vi "华为UPS2000-G获取UPS状态.vi"(8 "error in (no error)":errorcluster, 11 "MB session in":refnum<class "MB_Master.lvclass">) -> (0 "error out":errorcluster, 1 "UPS状态":bool[](array[boolean]), 2 "UPS参数":T1 {"开机状态" items=["关机", "开机中", "开机失败", "开机完成"]}, 3 "MB session out":refnum<class "MB_Master.lvclass">)   [LabVIEW 2016, in "环境动力监测库.lvlib" / "UPS库.lvlib"]
uses:
  <vilib>/Plasmionique/MB Master/MB_Master/MB_Master.lvclass
  <vilib>/Plasmionique/MB Master/MB Master.lvlib
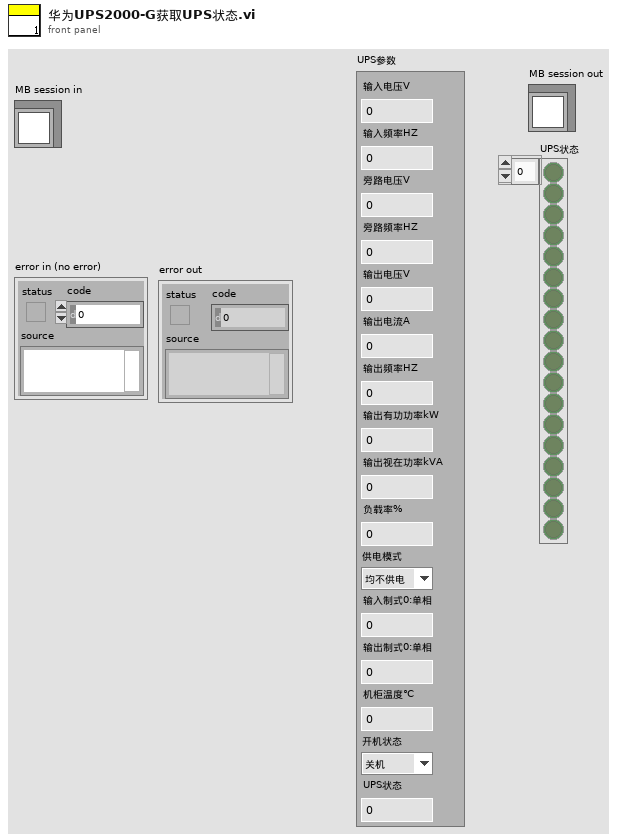
[diagram p1: front panel]
types:
  T1 = cluster{"输入电压V":dbl, "输入频率HZ":dbl, "旁路电压V":dbl, "旁路频率HZ":dbl, "输出电压V":dbl, "输出电流A":dbl, "输出频率HZ":dbl, "输出有功功率kW":dbl, "输出视在功率kVA":dbl, "负载率%":dbl, "供电模式":enum16{"均不供电", "旁路供电", "主路供电", "电池供电", "主路ECO"}, "输入制式0:单相":u16, "输出制式0:单相":u16, "机柜温度℃":dbl, "开机状态":u16, "UPS状态":u8}
  T2 = cluster{dbl, dbl, dbl, dbl, dbl, dbl, dbl, dbl, dbl, dbl, u16, u16, u16, dbl, u16, "元素":u16}
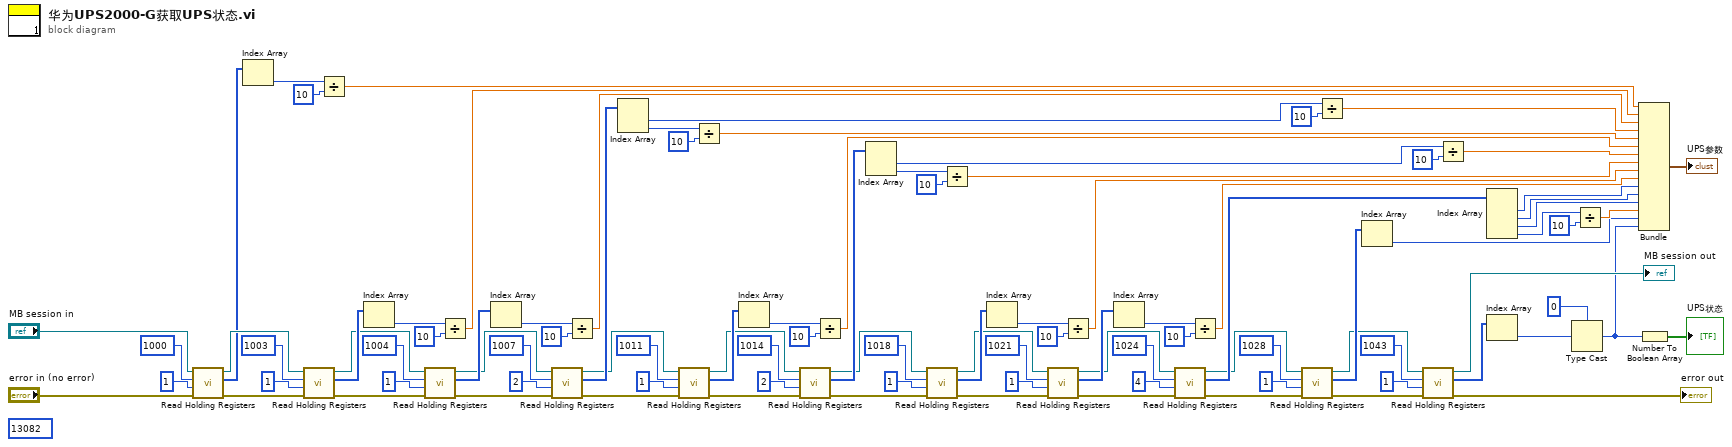
[diagram p0: block diagram]
diagram:
  (unwired) u16 13082 ("starting address")
  n1 = call <vilib>:"Read Holding Registers.vi"("error in (no error)"="error in (no error)", "quantity"=u16 1, "starting address"=u16 1000, "MB session in"="MB session in") -> ("error out"=w87:errorcluster, "Registers"=w93:u16[], "MB session out"=w96:refnum<class "MB_Master.lvclass">)  [unwired: 5 in]
  n2 = Index Array(array=w93) -> (element=w91:u16)  [unwired: 1 in]
  n3 = call <vilib>:"Read Holding Registers.vi"("error in (no error)"=w87, "quantity"=u16 1, "starting address"=u16 1003, "MB session in"=w96) -> ("error out"=w79:errorcluster, "Registers"=w84:u16[], "MB session out"=w80:refnum<class "MB_Master.lvclass">)  [unwired: 5 in]
  n4 = Divide(x=w91, y=u16 10) -> (x/y=w90:dbl)
  n5 = Index Array(array=w84) -> (element=w86:u16)  [unwired: 1 in]
  n6 = call <vilib>:"Read Holding Registers.vi"("error in (no error)"=w79, "quantity"=u16 1, "starting address"=u16 1004, "MB session in"=w80) -> ("error out"=w71:errorcluster, "Registers"=w76:u16[], "MB session out"=w72:refnum<class "MB_Master.lvclass">)  [unwired: 5 in]
  n7 = Divide(x=w86, y=u16 10) -> (x/y=w83:dbl)
  n8 = Index Array(array=w76) -> (element=w77:u16)  [unwired: 1 in]
  n9 = call <vilib>:"Read Holding Registers.vi"("error in (no error)"=w71, "quantity"=u16 2, "starting address"=u16 1007, "MB session in"=w72) -> ("error out"=w60:errorcluster, "Registers"=w68:u16[], "MB session out"=w61:refnum<class "MB_Master.lvclass">)  [unwired: 5 in]
  n10 = Divide(x=w77, y=u16 10) -> (x/y=w75:dbl)
  n11 = Index Array(array=w68) -> (element #1=w70:u16, element #2=w66:u16)  [unwired: 2 in]
  n12 = call <vilib>:"Read Holding Registers.vi"("error in (no error)"=w60, "quantity"=u16 1, "starting address"=u16 1011, "MB session in"=w61) -> ("error out"=w52:errorcluster, "Registers"=w57:u16[], "MB session out"=w53:refnum<class "MB_Master.lvclass">)  [unwired: 5 in]
  n13 = Divide(x=w66, y=u16 10) -> (x/y=w64:dbl)
  n14 = Index Array(array=w57) -> (element=w59:u16)  [unwired: 1 in]
  n15 = call <vilib>:"Read Holding Registers.vi"("error in (no error)"=w52, "quantity"=u16 2, "starting address"=u16 1014, "MB session in"=w53) -> ("error out"=w41:errorcluster, "Registers"=w50:u16[], "MB session out"=w42:refnum<class "MB_Master.lvclass">)  [unwired: 5 in]
  n16 = Divide(x=w59, y=u16 10) -> (x/y=w56:dbl)
  n17 = Index Array(array=w50) -> (element #1=w51:u16, element #2=w47:u16)  [unwired: 2 in]
  n18 = call <vilib>:"Read Holding Registers.vi"("error in (no error)"=w41, "quantity"=u16 1, "starting address"=u16 1018, "MB session in"=w42) -> ("error out"=w33:errorcluster, "Registers"=w39:u16[], "MB session out"=w35:refnum<class "MB_Master.lvclass">)  [unwired: 5 in]
  n19 = Divide(x=w47, y=u16 10) -> (x/y=w45:dbl)
  n20 = Index Array(array=w39) -> (element=w40:u16)  [unwired: 1 in]
  n21 = call <vilib>:"Read Holding Registers.vi"("error in (no error)"=w33, "quantity"=u16 1, "starting address"=u16 1021, "MB session in"=w35) -> ("error out"=w25:errorcluster, "Registers"=w31:u16[], "MB session out"=w26:refnum<class "MB_Master.lvclass">)  [unwired: 5 in]
  n22 = Divide(x=w40, y=u16 10) -> (x/y=w34:dbl)
  n23 = Index Array(array=w31) -> (element=w37:u16)  [unwired: 1 in]
  n24 = call <vilib>:"Read Holding Registers.vi"("error in (no error)"=w25, "quantity"=u16 4, "starting address"=u16 1024, "MB session in"=w26) -> ("error out"=w4:errorcluster, "Registers"=w24:u16[], "MB session out"=w8:refnum<class "MB_Master.lvclass">)  [unwired: 5 in]
  n25 = Divide(x=w37, y=u16 10) -> (x/y=w29:dbl)
  n26 = call <vilib>:"Read Holding Registers.vi"("error in (no error)"=w4, "quantity"=u16 1, "starting address"=u16 1028, "MB session in"=w8) -> ("error out"=w5:errorcluster, "Registers"=w9:u16[], "MB session out"=w7:refnum<class "MB_Master.lvclass">)  [unwired: 5 in]
  n27 = Divide(x=w70, y=u16 10) -> (x/y=w65:dbl)
  n28 = Index Array(array=w9) -> (element=w6:u16)  [unwired: 1 in]
  n29 = call <vilib>:"Read Holding Registers.vi"("error in (no error)"=w5, "quantity"=u16 1, "starting address"=u16 1043, "MB session in"=w7) -> ("error out"=→"error out":errorcluster, "Registers"=w14:u16[], "MB session out"=→"MB session out":refnum<class "MB_Master.lvclass">)  [unwired: 5 in]
  n30 = Divide(x=w51, y=u16 10) -> (x/y=w46:dbl)
  n31 = Index Array(array=w24) -> (element #1=w23:u16, element #2=w22:u16, element #3=w20:u16, element #4=w19:u16)  [unwired: 4 in]
  n32 = Index Array(array=w14) -> (element=w2:u16)  [unwired: 1 in]
  n33 = Type Cast(type=u16 0 ("元素"), x=w2) -> (*(type *) &x=w1:u16)
  n34 = Divide(x=w19, y=u16 10) -> (x/y=w18:dbl)
  n35 = Bundle(w90, w83, w75, w65, w64, w56, w46, w45, w34, w29, w23, w22, w20, w18, w6, "元素"=w1) -> (→"UPS参数":T2)  [unwired: 1 in]
  n36 = Number To Boolean Array(number=w1) -> (Boolean array=→"UPS状态":bool[])
